vi "History Write.vi"(4 "error in (no error)":errorcluster, 5 "Value":path[](array[path]), 6 "Container State":T2, 7 "Display State In":T1) -> (0 "error out":errorcluster, 3 "Display State Out":T1)   [LabVIEW 2009, in "HistoryPath.xctl"]
uses:
  HistoryPath.xctl
  <vilib>/_xctls/Container State.ctl
  State.ctl
  <vilib>/_xctls/XControlSupport.lvlib
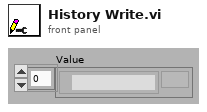
[diagram p1: front panel]
types:
  T1 = typedef "HistoryPath.xctl/State.ctl" = cluster{"History":path[], "History Length":i32}
  T2 = typedef "XControlSupport.lvlib/Container State.ctl" = cluster{"Indicator?":bool, "Run Mode?":bool, " Refnum":refnum<vi>}
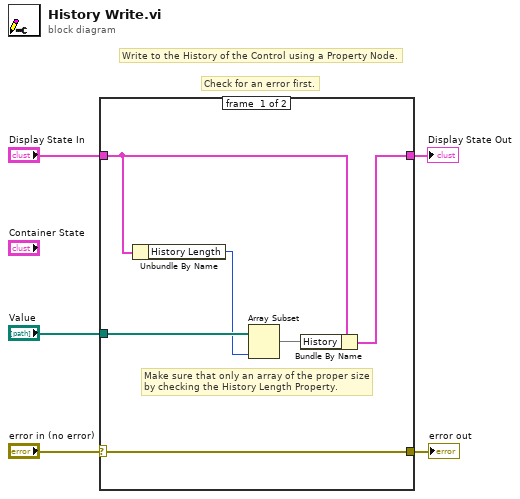
[diagram p0: block diagram]
diagram:
  # "Check for an error first."
  # "Write to the History of the Control using a Property Node."
  n1 = case shown="No Error" "error in (no error)" {
    selector: "error in (no error)" -> [w10 w13]
    tunnel: [w6 w12] -> w4
    tunnel: "Display State In" -> [w7 w12]
    tunnel: [w10 w13] -> w3
    tunnel: "Value" -> [w11 _]
    frame #0 {
      # "Make sure that only an array of the proper size\nby checking the History Length Property."
      n2 = Unbundle By Name(w7) -> ("History Length"=w8:i32)
      n3 = Array Subset(array=w11, length=w8) -> (w9:path[])  [unwired: 1 in]
      n4 = Bundle By Name(cluster=w7, "History"=w9) -> (w6:T1)
    }
    frame #1 {
    }
  }
  "error out" <- w3
  "Display State Out" <- w4
